vi "adam-4xxxl.vi"() -> ()   [LabVIEW 2024]
panel:
  in  "clear-command":bool
  in  "Channels":T1
  out "concatenated string":string
  in  "Single/Multi Channel":bool
  in  "Deliminator Char":string(combo)
  in  "Manual Command":string="#01"
  out "read buffer":string
  out "Bytes at Port":u32
  in  "send-command":bool
  out "Channel Number":string
  out "Channel State String":string
  out "Device Address":string
  in  "Device Address":i32=1 min=0 max=100 step=1
  in  "baud rate (19200)":u32=19200
  in  "COM Port (COM10)":refnum<visa-resource-name>="COM10"
  in  "Stop Program":bool
  out "command":string
  in  "Channel Number":i32=1 min=0 max=7 step=1
  in  "Channel State Bit":bool
  out "Bytes Written":u32
  out "error":errorcluster
  # "ADAM-4xxx Test VI"
  # "Set COM before  running"
  # "To Use, either:\n- Enter Manual Command in Text box\nOR\n- Set up command using options below\nThen:\n- Press Send Command"
  # "Example Commands:\n  Code   |    Behaviour       | Success | Failed \n---      |---                 |---      |---\nadam-4069 8x Power Relay\n#010000 \t| All Channels: Off  |\t   > \t  | ?AA \n#01000F \t| All Channels: On \t |         |\n#011000 \t| Channel 0: Off \t   |\t        |\n#011001 \t| Channel 0: On \t\t   |         |\n#011100 \t| Channel 1: Off \t\t  |         |\n#011101 \t| Channel 1: On \t    |         |"
  # "adam-4017+ 8x AI\nadam-4018+ 8x T/C & mA\n#01 \t    | All Channels: data |>+data+data...| ?AA \nAA = module address"
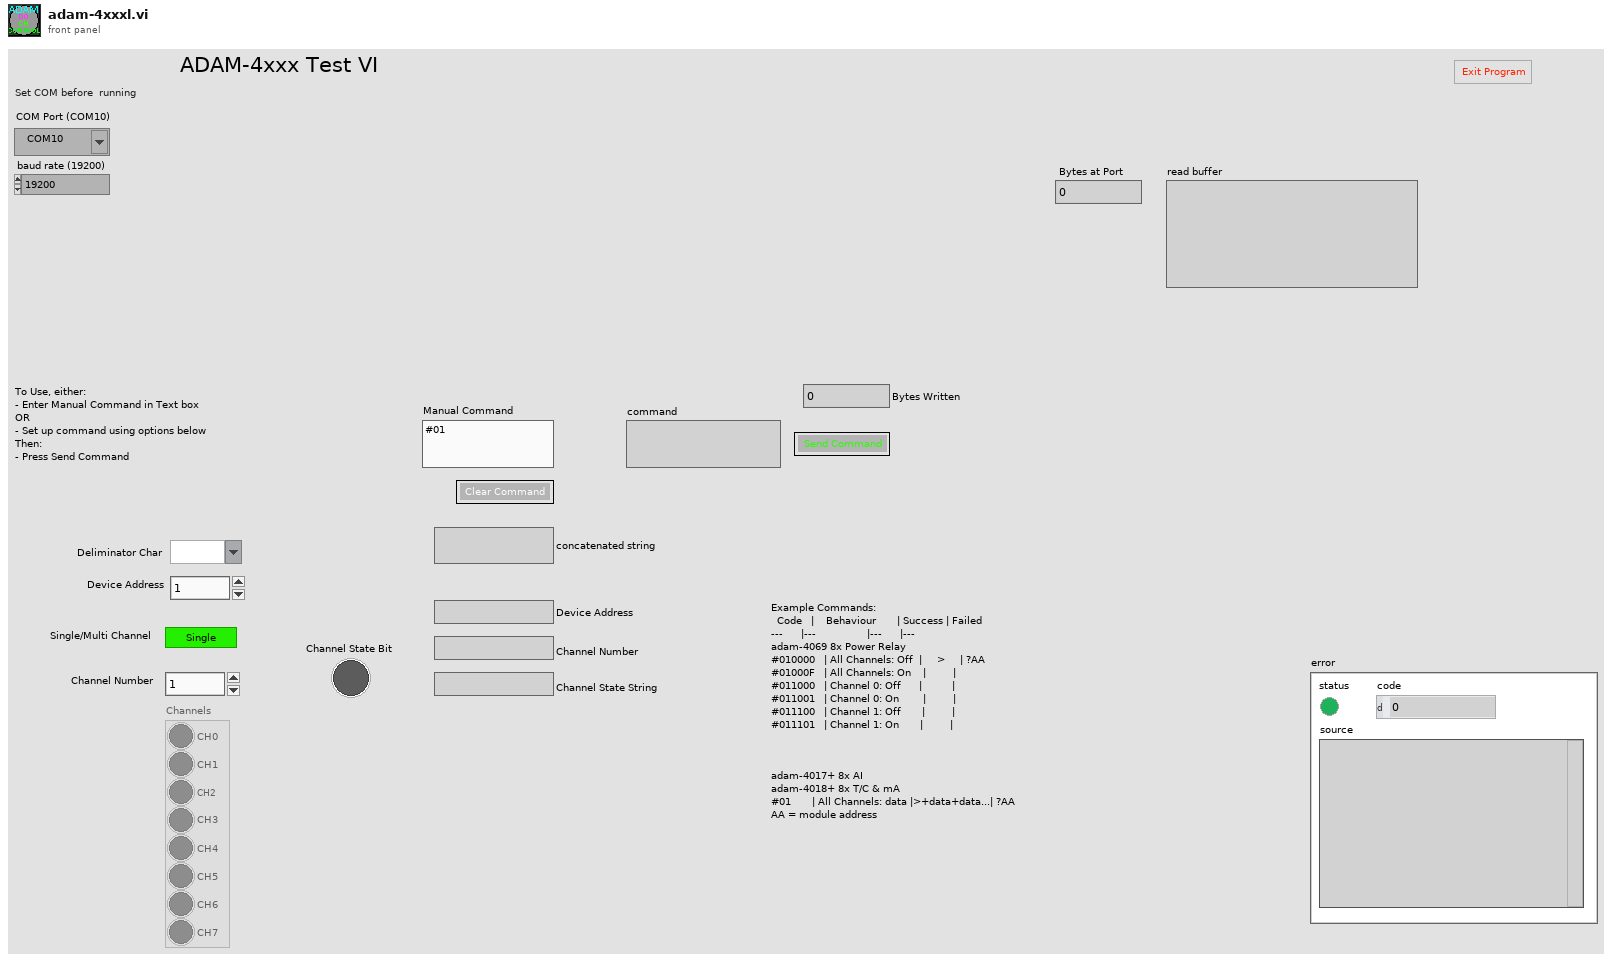
[diagram p1: front panel]
types:
  T1 = cluster{"CH0":bool, "CH1":bool, "CH2":bool, "CH3":bool, "CH4":bool, "CH5":bool, "CH6":bool, "CH7":bool}
  T2 = enum8{"Enabled", "Disabled", "Disabled and Grayed Out"}
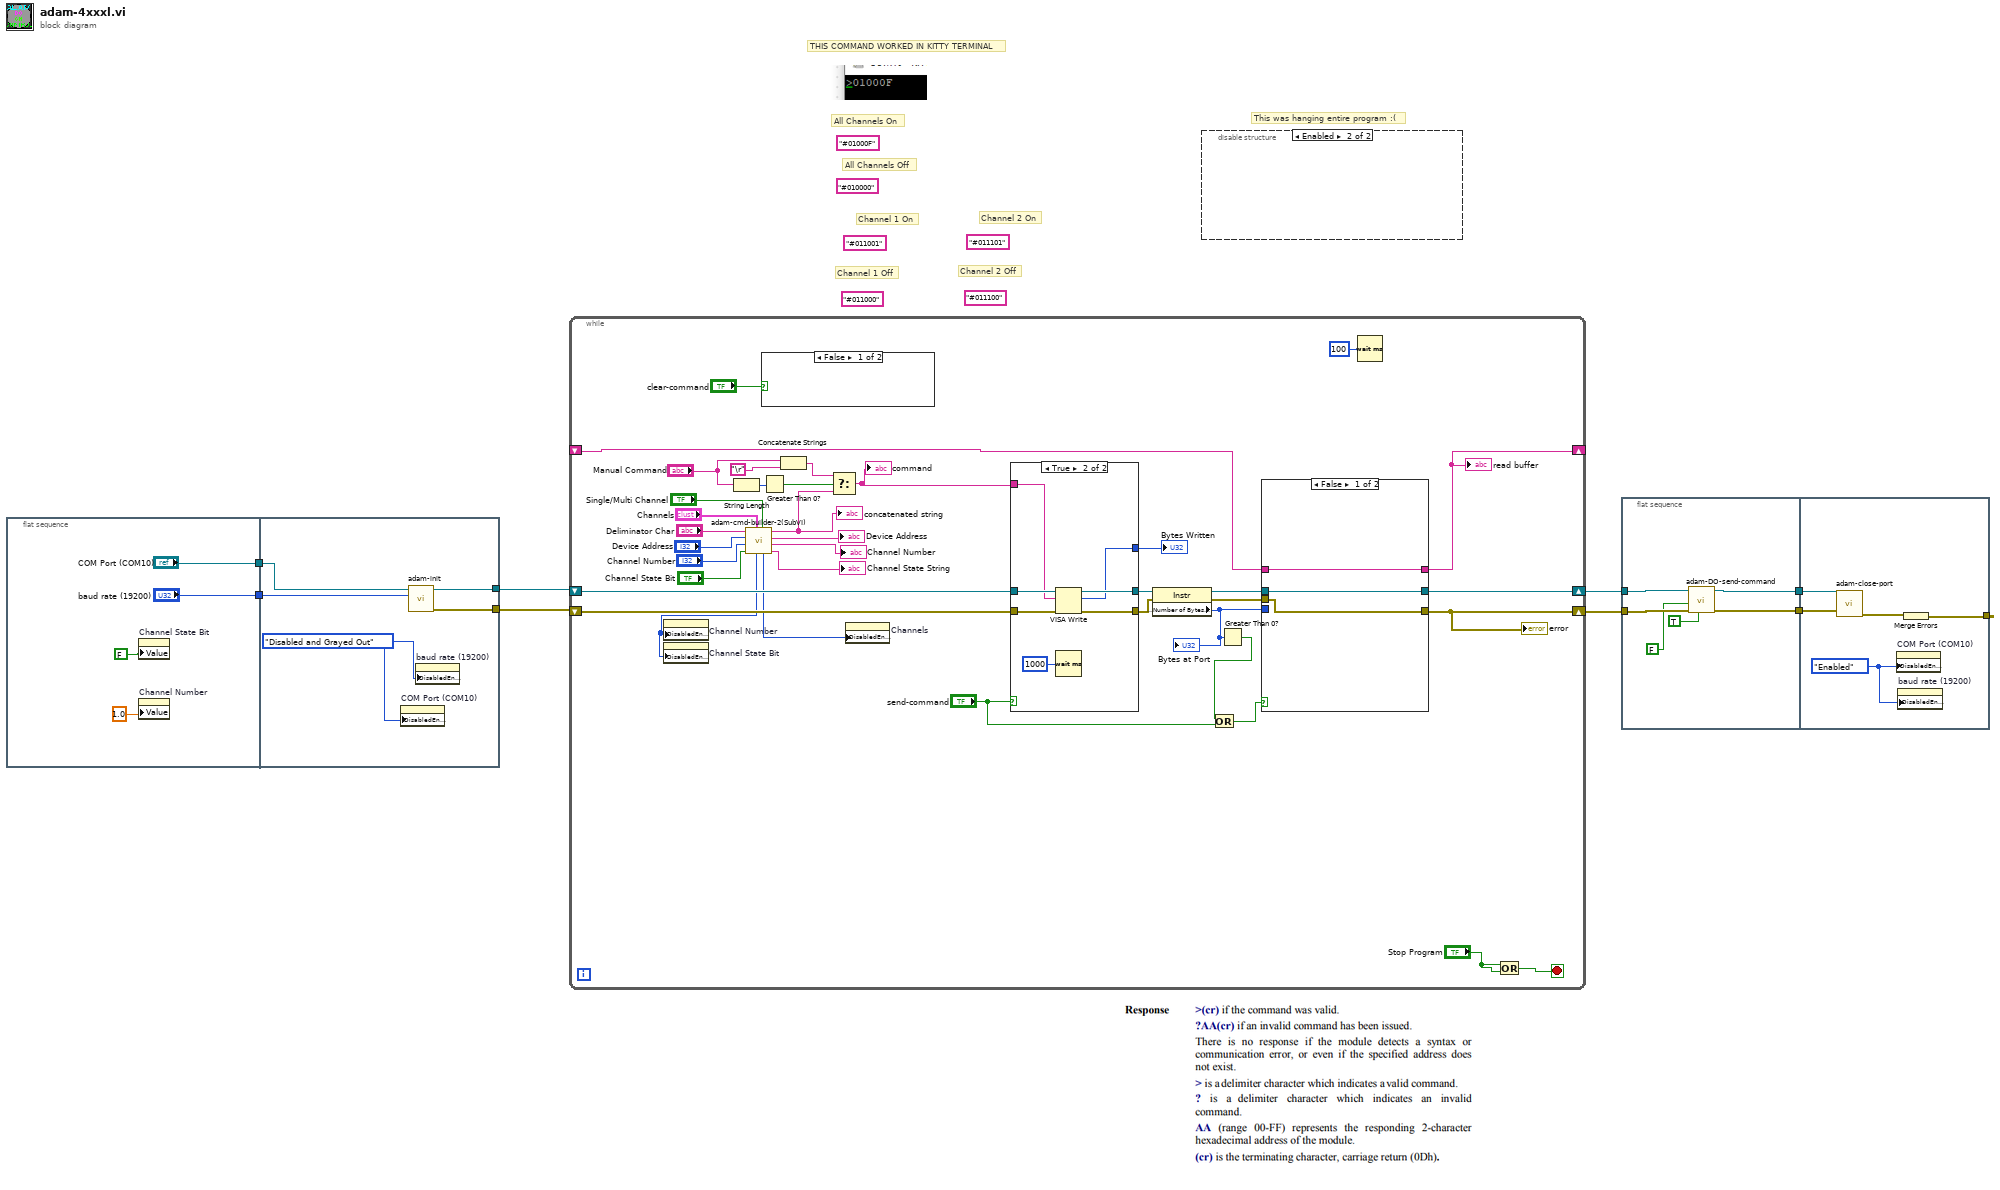
[diagram p0: block diagram]
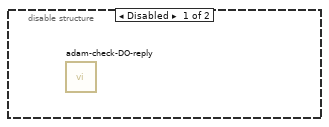
[diagram p2: hidden frame]
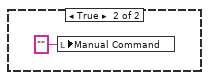
[diagram p3: hidden frame]
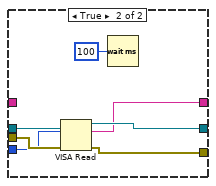
[diagram p4: hidden frame]
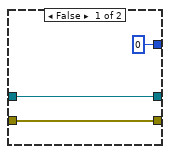
[diagram p5: hidden frame]
diagram:
  (unwired) "#011101" ("write buffer")
  (unwired) "#011100" ("write buffer")
  (unwired) "#011001" ("write buffer")
  (unwired) "#011000" ("write buffer")
  (unwired) "#010000" ("write buffer")
  (unwired) "#01000F" ("write buffer")
  # "This was hanging entire program :("
  # "Channel 2 Off"
  # "Channel 2 On"
  # "Channel 1 Off"
  # "Channel 1 On"
  # "All Channels Off"
  # "All Channels On"
  # "THIS COMMAND WORKED IN KITTY TERMINAL"
  n1 = flat-sequence {
    tunnel: ["baud rate (19200)"] -> w2
    tunnel: ["COM Port (COM10)"] -> w1
    tunnel: [w17] -> w6
    tunnel: [w16] -> w5
    tunnel: w2 -> [w15]
    tunnel: w1 -> [w14]
    frame #0 {
      n2 = property on="Channel State Bit" class="Bool (strict)"("Value"=FALSE ("Channel Active")) -> ()  [unwired: 2 in, 2 out]
      n3 = property on="Channel Number" class="DigNum (strict)"("Value"=1.0 ("Channel Number")) -> ()  [unwired: 2 in, 2 out]
    }
    frame #1 {
      w13 = T2."Disabled and Grayed Out" ("Disabled")
      n4 = property on="COM Port (COM10)" class="VISAName"("DisabledEnum"=w13) -> ()  [unwired: 2 in, 2 out]
      n5 = call "adam-init.vi"("baud rate (19200)"=w15, "COM Port (COM10)"=w14) -> ("error out"=w16:errorcluster, "VISA resource name out"=w17:refnum<visa-resource-name>)  [unwired: 8 in]
      n6 = property on="baud rate (19200)" class="DigNum (strict)"("DisabledEnum"=w13) -> ()  [unwired: 2 in, 2 out]
    }
  }
  n7 = while {
    shift-right: [w43] -> w7
    shift-left: w6 -> [w52]
    shift-right: [w26] -> w8
    shift-left: w5 -> [w51]
    shift-right: [w42] -> _
    shift-left: _ -> [w41]
    stop <- w54 stop-if-true
    n8 = String Length(string="Manual Command") -> (length=w40:i32)
    n9 = call "adam-cmd-builder-2(SubVI).vi"("Single/Multi Channel"="Single/Multi Channel", "Channels"="Channels", "Channel State Bit"="Channel State Bit", "Channel Number in"="Channel Number", "Device Address in"="Device Address", "Deliminator Char"="Deliminator Char") -> ("Channel State String"=→"Channel State String":string, "Channel Number out"=→"Channel Number":string, "Device Address out"=→"Device Address":string, "concatenated string"=w30:string, "MultiCH-enable"=w31:T2, "SingleCH-enable"=w32:T2)
    "concatenated string" <- w30
    n10 = property on="Channel Number" class="DigNum (strict)"("DisabledEnum"=w32) -> ()  [unwired: 2 in, 2 out]
    n11 = property on="Channel State Bit" class="Bool (strict)"("DisabledEnum"=w32) -> ()  [unwired: 2 in, 2 out]
    n12 = case shown="False" "clear-command" {
      frame False {
      }
      frame True {
        n13 = local write "Manual Command"("" ("Manual Command")) -> ()
      }
    }
    n14 = Greater Than 0?(x=w40) -> (x > 0?=w39:bool)
    n15 = Concatenate Strings("Manual Command", "\r") -> (w21:string)
    n16 = Select(t=w21, s=w39, f=w30) -> (s? t:f=w18:string)
    "command" <- w18
    n17 = property on="Channels" class="Clust (strict)"("DisabledEnum"=w31) -> ()  [unwired: 2 in, 2 out]
    n18 = case shown="True" "send-command" {
      tunnel: w52 -> [w67 w75]
      tunnel: w51 -> [w66 w74]
      tunnel: [w66 w73] -> w47
      tunnel: [w67 w72] -> w48
      tunnel: [u32 0 ("return count") w71] -> w50
      tunnel: w18 -> [_ w70]
      frame False {
      }
      frame True {
        n19 = VISA Write(VISA resource name=w75, write buffer=w70, error in (no error)=w74) -> (VISA resource name out=w72:refnum<visa-resource-name>, return count=w71:u32, error out=w73:errorcluster)
        n20 = Wait (ms)(milliseconds to wait=u32 1000) -> ()  [unwired: 1 out]
      }
    }
    "Bytes Written" <- w50
    n21 = property class="Instr"(reference=w48, error in=w47) -> (reference out=w45:refnum<visa-resource-name>, error out=w46:errorcluster, "Serial Settings:Number of Bytes at Serial Port"=w44:u32)
    "Bytes at Port" <- w44
    n22 = Greater Than 0?(x=w44) -> (x > 0?=w25:bool)
    n23 = Or(x=w25, y="send-command") -> (x .or. y?=w23:bool)
    n24 = case shown="False" w23 {
      tunnel: w46 -> [w57 w64]
      tunnel: w45 -> [w58 w65]
      tunnel: w44 -> [_ w63]
      tunnel: [w58 w62] -> w43
      tunnel: [w57 w61] -> w26
      tunnel: [w56 w60] -> w42
      tunnel: w41 -> [w56 _]
      frame False {
      }
      frame True {
        n25 = VISA Read(VISA resource name=w65, byte count=w63, error in (no error)=w64) -> (VISA resource name out=w62:refnum<visa-resource-name>, read buffer=w60:string, error out=w61:errorcluster)  [unwired: 1 out]
        n26 = Wait (ms)(milliseconds to wait=u32 100) -> ()  [unwired: 1 out]
      }
    }
    "read buffer" <- w42
    "error" <- w26
    n27 = Wait (ms)(milliseconds to wait=u32 100) -> ()  [unwired: 1 out]
    n28 = Or(x="Stop Program", y="Stop Program") -> (x .or. y?=w54:bool)
  }
  n29 = disable-structure shown="Enabled" {
    frame Disabled {
      n30 = call "adam-check-DO-reply.vi"() -> ()  [unwired: 7 in, 5 out]
    }
    frame Enabled {
    }
  }
  n31 = flat-sequence {
    tunnel: w8 -> [w81]
    tunnel: w7 -> [w77]
    tunnel: [w80] -> w4
    tunnel: [w78] -> w3
    tunnel: w4 -> [w84]
    tunnel: w3 -> [w85]
    tunnel: [w83] -> _
    frame #0 {
      n32 = call "adam-DO-send-command.vi"("Stop All"=TRUE, "error in (no error)"=w81, "Channel Active"=FALSE, "VISA Refnum in"=w77) -> ("error out"=w78:errorcluster, "VISA Refnum out"=w80:refnum<visa-resource-name>)  [unwired: 2 in, 4 out]
    }
    frame #1 {
      w82 = T2."Enabled" ("Disabled")
      n33 = call "adam-close-port.vi"("error in (no error)"=w85, "VISA Refnum in"=w84) -> ("error out"=w86:errorcluster)  [unwired: 9 in]
      n34 = property on="COM Port (COM10)" class="VISAName"("DisabledEnum"=w82) -> ()  [unwired: 2 in, 2 out]
      n35 = property on="baud rate (19200)" class="DigNum (strict)"("DisabledEnum"=w82) -> ()  [unwired: 2 in, 2 out]
      n36 = Merge Errors(w86) -> (w83:errorcluster)
    }
  }
